vi "ChassisSystem.vi"(1 "Targets":dbl[](array[numeric]), 2 "Robot Maximum Rate":dbl, 3 "PID constants":dbl[](array[numeric]), 4 "Gyro and Accelerometer reference names":string[](array[string]), 5 "Encoder Reference names":string[](array[string]), 6 "Motor and PWM reference names":string[](array[string])) -> (0 "Reported Status":T1 {"Rotation Status" items=["no Rotation motor output", "Rotate Right", "Rotate Left"]; "X status" items=["no X motor output", "Strafe Right", "Strafe Left"]; "Y status" items=["no Y motor output", "Drive Forward", "Drive Backward"]})   [LabVIEW 2014]
uses:
  <vilib>/Rock Robotics/WPI/RobotDrive/WPI_RobotDriveGetSetRefNum.vi
panel:
  # "These are read from the joystick"
  # "X target"
  # "Y target"
  # "Rotation Target"
  # "Front Left Encoder"
  # "Front Right Encoder"
  # "Rear Left Encoder"
  # "Rear Right Encoder"
  # "Robot Drive"
  # "Front Left Motor"
  # "Front Right Motor"
  # "Rear Left Motor"
  # "Rear Right Motor"
  # "Gyro"
  # "Accelerometer"
  # "P"
  # "I"
  # "D"
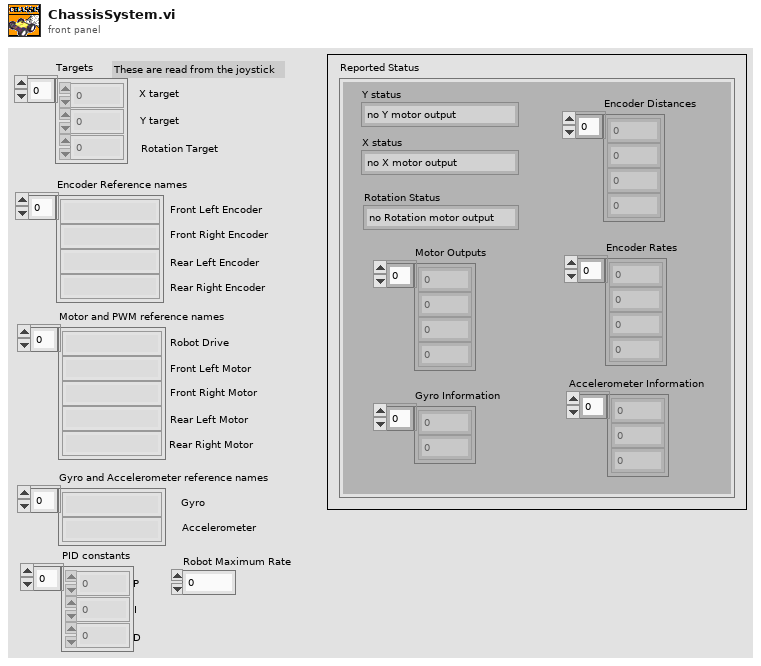
[diagram p1: front panel]
types:
  T1 = cluster{"Y status":u16, "X status":u16, "Rotation Status":u16, "Motor Outputs":dbl[], "Encoder Distances":dbl[], "Encoder Rates":dbl[], "Gyro Information":dbl[], "Accelerometer Information":dbl[]}
  T2 = typedef "WPI_GyroDevRef.ctl" = cluster{"DevStatus":errorcluster, "Analog Module":T3, "Analog Channel":T4, "Offset":dbl, "Gain (VoltsPerDegree/Second)":dbl}
  T3 = typedef "FPGA_TypedefAnalogModule.ctl" = enum16{"Controller 1"}
  T4 = typedef "FPGA_AIChannel.ctl" = enum8{"AI 0", "AI 1", "AI 2", "AI 3", "AI MXP 0", "AI MXP 1", "AI MXP 2", "AI MXP 3", "Invalid"}
  T5 = typedef "WPI_AccelerometerDevRef.ctl" = cluster{"DevStatus":errorcluster, "Controller":T3, "Scaling":T6, "Analog Channels":T7, "I2C Bus":T8, "SPI Bus":T9, "Accel Range":T10, "ADXL345 Axes":T11, "Handle":i32, "Device Address":u8, "Accel Type":enum16{"Analog", "ADXL345 I2C", "ADXL345 SPI", "Internal"}}
  T6 = typedef "WPI_AccelerometerScaling.ctl" = cluster{"Gain (VoltsPerG)":dbl, "Center Voltage":dbl}
  T7 = typedef "WPI_AccelerometerAnalogChannels.ctl" = cluster{"X-Axis":T4, "Y-Axis":T4, "Z-Axis":T4}
  T8 = typedef "i2c_bus.ctl" = enum16{"I2C On-Board", "I2C MXP", "Invalid"}
  T9 = typedef "spi_bus.ctl" = enum16{"SPI On-Board, CS0", "SPI On-Board, CS1", "SPI On-Board, CS2", "SPI On-Board, CS3", "SPI MXP", "Invalid"}
  T10 = typedef "ADXL345 Range.ctl" = u8
  T11 = typedef "WPI_AccelerometerADXL345 Axes.ctl" = cluster{"X-Axis":bool, "Y-Axis":bool, "Z-Axis":bool}
  T12 = cluster{"X-Axis":dbl, "Y-Axis":dbl, "Z-Axis":dbl}
  T13 = typedef "WPI_EncoderDevRef.ctl" = cluster{"DevStatus":errorcluster, "EncoderIndex":T14, "CounterIndex":T15, "DistancePerCount":dbl, "Decoding Type":T16}
  T14 = typedef "FPGA_EncoderIdx.ctl" = enum8{"Enc 0", "Enc 1", "Enc 2", "Enc 3", "Enc 4", "Enc 5", "Enc 6", "Enc 7", "Invalid"}
  T15 = typedef "FPGA_CounterCtrSystemIndex.ctl" = enum8{"Ctr 0", "Ctr 1", "Ctr 2", "Ctr 3", "Ctr 4", "Ctr 5", "Ctr 6", "Ctr 7", "Invalid"}
  T16 = typedef "WPI_EncoderType.ctl" = enum16{"1x", "2x", "4x"}
  T17 = typedef "WPI_RobotDriveDevRef.ctl" = cluster{"DevStatus":errorcluster, "Motors[]":T18[], "Square Inputs":bool, "Max Output":dbl}
  T18 = typedef "WPI_MotorControlDeviceRef.ctl" = cluster{"DeviceStatus":errorcluster, "Type":T19, "PWM":cluster{"Controller":T20, "PWM Channel":T21, "DeadBand":T22}, "CAN":cluster{"Device Number":u8, "Control Mode":T23, "Semaphore":T24, "Max Vout":dbl, "TalonSRX Control Mode":T25}, "Invert":bool, "TransformRef":T26, "InvTransformRef":T26}
  T19 = typedef "WPI_MotorControlType.ctl" = enum16{"PWM", "CAN", "CANTalonSRX"}
  T20 = typedef "FPGA_TypedefDigitalModule.ctl" = enum16{"Controller 1"}
  T21 = typedef "FPGA_DIOPWMChannel.ctl" = enum8{"PWM 0", "PWM 1", "PWM 2", "PWM 3", "PWM 4", "PWM 5", "PWM 6", "PWM 7", "PWM 8", "PWM 9", "PWM MXP 0", "PWM MXP 1", "PWM MXP 2", "PWM MXP 3", "PWM MXP 4", "PWM MXP 5", "PWM MXP 6", "PWM MXP 7", "PWM MXP 8", "PWM MXP 9", "Invalid"}
  T22 = typedef "WPI_PWMDeadband.ctl" = cluster{"Name":string, "maxPositivePwm":i32, "minPositivePwm":i32, "centerPwm":i32, "maxNegativePwm":i32, "minNegativePwm":i32, "angularRange":u16}
  T23 = typedef "WPI_CANJaguar_ControlMode.ctl" = enum8{"Percent VBus", "Current", "Speed", "Position", "Voltage"}
  T24 = typedef "Semaphore RefNum" = refnum<k1>
  T25 = typedef "WPI_CANTalonSRX_APIControlMode.ctl" = enum8{"Percent VBus", "Speed", "Position", "Slave", "Unchanged / Invalid"}
  T26 = typedef "WPI_PWMTransform_ConPane.ctl" = refnum<vi>
  T27 = typedef "WPI_CANTalonSRX_GlobalStatus.ctl" = cluster{"Applied Throttle":dbl, "Module Enabled":bool, "CAN Error":errorcluster, "Closed Loop Error":dbl, "Forward Limit Switch Closed":bool, "Reverse Limit Switch Closed":bool, "Sensor Position":dbl, "Sensor Velocity":dbl, "Current":dbl, "Sticky Fault - Over Temp":bool, "Sticky Fault - Under Voltage":bool, "Sticky Fault - Forward Limit":bool, "Sticky Fault - Reverse Limit":bool, "Sticky Fault - Forward Soft Limit":bool, "Sticky Fault - Reverse Soft Limit":bool, "Brake is Enabled":bool, "Encoder Position":dbl, "Encoder Velocity":dbl, "Encoder Index Count":dbl, "Encoder A Pin State":bool, "Encoder B Pin State":bool, "Encoder Index Pin State":bool, "Analog In":dbl, "Analog In Velocity":dbl, "Temperature (C)":dbl, "Battery Voltage":dbl}
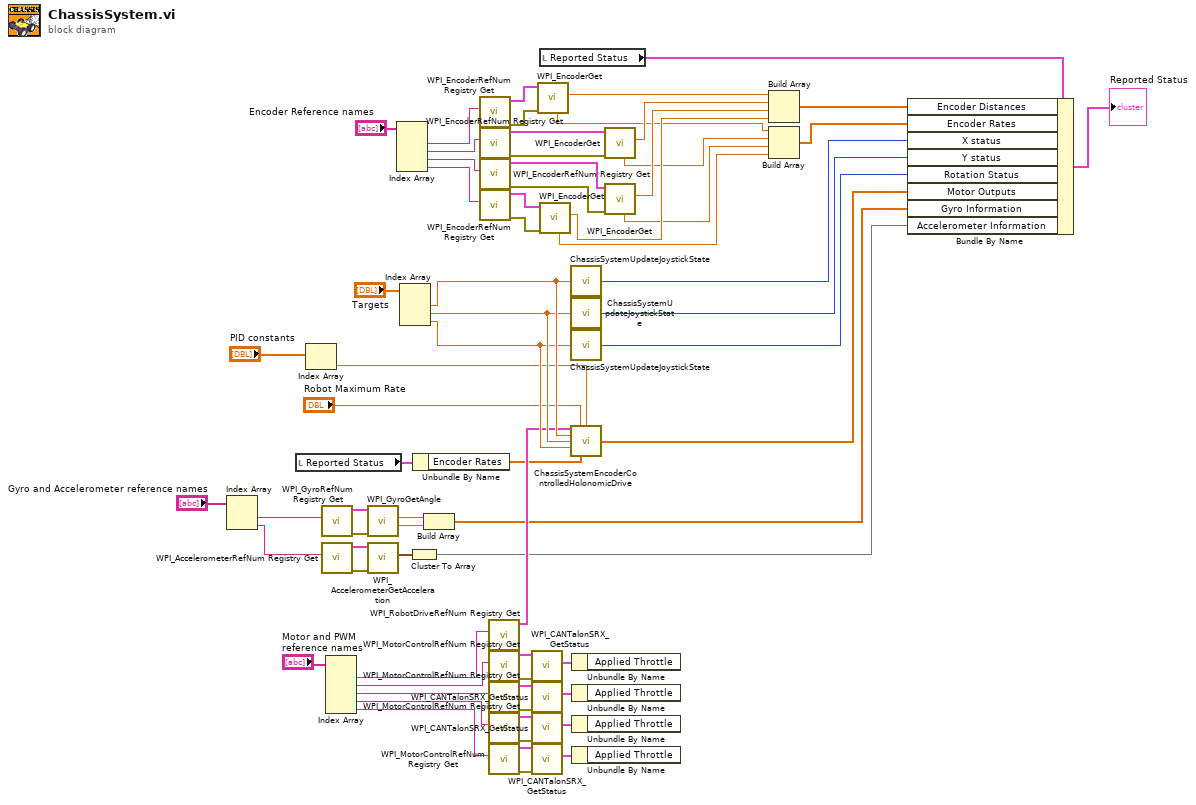
[diagram p0: block diagram]
diagram:
  n1 = Index Array(array="Gyro and Accelerometer reference names") -> (element #1=w11:string, element #2=w5:string)  [unwired: 2 in]
  n2 = local read "Reported Status"() -> (w18:T1)
  n3 = Index Array(array="PID constants") -> (element=w13:dbl)  [unwired: 1 in]
  n4 = call <vilib>:"WPI_GyroRefNum Registry Get.vi"("refnum name"=w11) -> ("error out"=w10:errorcluster, "GyroDevRef"=w9:T2)  [unwired: 9 in]
  n5 = call <vilib>:"WPI_AccelerometerRefNum Registry Get.vi"("refnum name"=w5) -> ("error out"=w4:errorcluster, "AccelerometerDevRef"=w3:T5)  [unwired: 9 in]
  n6 = Index Array(array="Motor and PWM reference names") -> (element #1=w66:string, element #2=w65:string, element #3=w64:string, element #4=w63:string, element #5=w62:string)  [unwired: 5 in]
  n7 = call <vilib>:"WPI_GyroGetAngle.vi"("error in (no error)"=w10, "GyroDevRef"=w9) -> ("Angular Rate"=w7:dbl, "Angle"=w8:dbl)  [unwired: 6 in, 2 out]
  n8 = call <vilib>:"WPI_AccelerometerGetAcceleration.vi"("error in"=w4, "AccelerometerDevRef"=w3) -> ("Accelerations"=w2:T12)  [unwired: 7 in, 2 out]
  n9 = Index Array(array="Encoder Reference names") -> (element #1=w68:string, element #2=w49:string, element #3=w47:string, element #4=w48:string)  [unwired: 4 in]
  n10 = Index Array(array="Targets") -> (element #1=w22:dbl, element #2=w21:dbl, element #3=w20:dbl)  [unwired: 3 in]
  n11 = Cluster To Array(cluster=w2) -> (array=w1:dbl[])
  n12 = Unbundle By Name(w18) -> ("Encoder Rates"=w17:dbl[])
  n13 = Build Array(w8, w7) -> (w6:dbl[])
  n14 = call <vilib>:"WPI_EncoderRefNum Registry Get.vi"("refnum name"=w68) -> ("error out"=w46:errorcluster, "EncoderDevRef"=w45:T13)  [unwired: 9 in]
  n15 = call <vilib>:"WPI_EncoderRefNum Registry Get.vi"("refnum name"=w49) -> ("error out"=w44:errorcluster, "EncoderDevRef"=w43:T13)  [unwired: 9 in]
  n16 = call <vilib>:"WPI_EncoderRefNum Registry Get.vi"("refnum name"=w47) -> ("error out"=w42:errorcluster, "EncoderDevRef"=w41:T13)  [unwired: 9 in]
  n17 = call <vilib>:"WPI_EncoderRefNum Registry Get.vi"("refnum name"=w48) -> ("error out"=w40:errorcluster, "EncoderDevRef"=w39:T13)  [unwired: 9 in]
  n18 = call <vilib>:"WPI_RobotDriveRefNum Registry Get.vi"("refnum name"=w66) -> ("RobotDriveDevRef"=w19:T17)  [unwired: 9 in, 1 out]
  n19 = call <vilib>:"WPI_MotorControlRefNum Registry Get.vi"("refnum name"=w65) -> ("error out"=w61:errorcluster, "MotorControlDevRef"=w60:T18)  [unwired: 9 in]
  n20 = call <vilib>:"WPI_MotorControlRefNum Registry Get.vi"("refnum name"=w64) -> ("error out"=w56:errorcluster, "MotorControlDevRef"=w57:T18)  [unwired: 9 in]
  n21 = call <vilib>:"WPI_MotorControlRefNum Registry Get.vi"("refnum name"=w63) -> ("error out"=w53:errorcluster, "MotorControlDevRef"=w54:T18)  [unwired: 9 in]
  n22 = call <vilib>:"WPI_MotorControlRefNum Registry Get.vi"("refnum name"=w62) -> ("error out"=w50:errorcluster, "MotorControlDevRef"=w51:T18)  [unwired: 9 in]
  n23 = call <vilib>:"WPI_CANTalonSRX_GetStatus.vi"("error in (no error)"=w61, "CAN Talon SRX Ref"=w60) -> ("Talon SRX Status"=w59:T27)  [unwired: 7 in, 2 out]
  n24 = call <vilib>:"WPI_CANTalonSRX_GetStatus.vi"("error in (no error)"=w56, "CAN Talon SRX Ref"=w57) -> ("Talon SRX Status"=w58:T27)  [unwired: 7 in, 2 out]
  n25 = call <vilib>:"WPI_CANTalonSRX_GetStatus.vi"("error in (no error)"=w53, "CAN Talon SRX Ref"=w54) -> ("Talon SRX Status"=w55:T27)  [unwired: 7 in, 2 out]
  n26 = call <vilib>:"WPI_CANTalonSRX_GetStatus.vi"("error in (no error)"=w50, "CAN Talon SRX Ref"=w51) -> ("Talon SRX Status"=w52:T27)  [unwired: 7 in, 2 out]
  n27 = call <vilib>:"WPI_EncoderGet.vi"("error in (no error)"=w46, "EncoderDevRef"=w45) -> ("Distance"=w37:dbl, "Rate"=w31:dbl)  [unwired: 4 in, 4 out]
  n28 = local read "Reported Status"() -> (w38:T1)
  n29 = call <vilib>:"WPI_EncoderGet.vi"("error in (no error)"=w40, "EncoderDevRef"=w39) -> ("Distance"=w34:dbl, "Rate"=w28:dbl)  [unwired: 4 in, 4 out]
  n30 = call "ChassisSystemUpdateJoystickState.vi"("Joystick Axis Value"=w22) -> ("Ring Output Status"=w25:i32)
  n31 = call "ChassisSystemUpdateJoystickState.vi"("Joystick Axis Value"=w21) -> ("Ring Output Status"=w24:i32)
  n32 = call "ChassisSystemUpdateJoystickState.vi"("Joystick Axis Value"=w20) -> ("Ring Output Status"=w23:i32)
  n33 = call "ChassisSystemEncoderControlledHolonomicDrive.vi"("RobotDriveDevRef"=w19, "Robot Maximum Rate"="Robot Maximum Rate", "Proportional Constant"=w13, "X"=w22, "Y"=w21, "Rotation"=w20, "Encoder Readings"=w17) -> ("Motor Values"=w16:dbl[])  [unwired: 6 in, 2 out]
  n34 = Unbundle By Name(w59) -> ()  [unwired: 1 out]
  n35 = Unbundle By Name(w58) -> ()  [unwired: 1 out]
  n36 = Unbundle By Name(w55) -> ()  [unwired: 1 out]
  n37 = Unbundle By Name(w52) -> ()  [unwired: 1 out]
  n38 = call <vilib>:"WPI_EncoderGet.vi"("error in (no error)"=w44, "EncoderDevRef"=w43) -> ("Distance"=w36:dbl, "Rate"=w30:dbl)  [unwired: 4 in, 4 out]
  n39 = call <vilib>:"WPI_EncoderGet.vi"("error in (no error)"=w42, "EncoderDevRef"=w41) -> ("Distance"=w35:dbl, "Rate"=w29:dbl)  [unwired: 4 in, 4 out]
  n40 = Build Array(w37, w36, w35, w34) -> (w33:dbl[])
  n41 = Build Array(w31, w30, w29, w28) -> (w27:dbl[])
  n42 = Bundle By Name(cluster=w38, "Encoder Distances"=w33, "Encoder Rates"=w27, "X status"=w25, "Y status"=w24, "Rotation Status"=w23, "Motor Outputs"=w16, "Gyro Information"=w6, "Accelerometer Information"=w1) -> (→"Reported Status":T1)
